vi "Remove Empty Keys.vi"(11 "Keyed Array":T1) -> (3 "Keyed Array":T1)   [LabVIEW 2014, in "Tools_KeyedArray.lvlib"]
uses:
  Tools_KeyedArray.lvlib
  KeyedArray.ctl
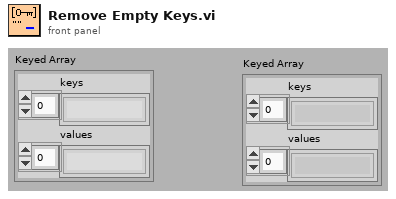
[diagram p1: front panel]
types:
  T1 = typedef "Tools_KeyedArray.lvlib/KeyedArray.ctl" = cluster{"keys":string[], "values":string[]}
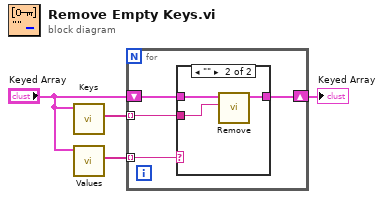
[diagram p0: block diagram]
diagram:
  n1 = call "Keys.vi"("array in"="Keyed Array") -> ("keys"=w2:string[])  [unwired: 6 out]
  n2 = call "Values.vi"("array in"="Keyed Array") -> ("values"=w3:string[])  [unwired: 6 out]
  n3 = for {
    shift-right: [w7] -> w1
    shift-left: "Keyed Array" -> [w8]
    tunnel: w3 -> [w6] mode=indexing
    tunnel: w2 -> [w5] mode=indexing
    n4 = case shown="\"\"" w6 {
      tunnel: [w9 w10] -> w7
      tunnel: w8 -> [w9 w12]
      tunnel: w5 -> [_ w11]
      frame Default {
      }
      frame "" {
        n5 = call "Remove.vi"("key"=w11, "array in"=w12) -> ("array out"=w10:T1)  [unwired: 1 in, 4 out]
      }
    }
  }
  "Keyed Array" <- w1
